vi "Choose_Device.vi"(3 "error in (no error)":errorcluster, 4 "Choose_Device":T1(ring), 5 "Index":i32) -> (0 "error out":errorcluster, 1 "Device_type":T1(ring), 2 "Index_Out":i32)   [LabVIEW 2013, in "FEMTO_LUCI-10.lvlib"]
doc: "This function sets the selected device."
uses:
  FEMTO_LUCI-10.lvlib
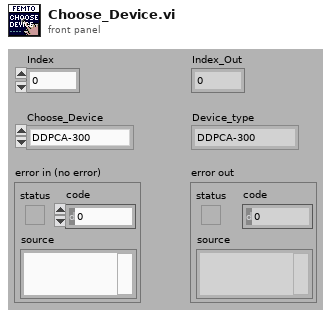
[diagram p1: front panel]
types:
  T1 = enum16{"DDPCA-300", "DLPCA-200", "DHPCA-100", "OE-200", "LIA-MV-150-S", "LIA-MV-150-D", "LIA-MV-200-L", "LIA-MV-200-H", "LIA-MVD-200-L", "LIA-MVD-200-H", "DLPVA-100-BUN-S", "DLPVA-100-BLN-S", "DLPVA-100-B-S", "DLPVA-100-B-D", "DLPVA-100-F-S", "DLPVA-100-F-D", "DHPVA-100", "DHPVA-200", "DUPVA-1-60", "DUPVA-1-70"}
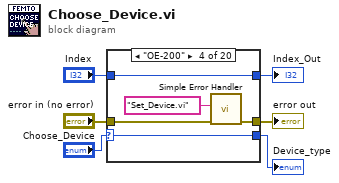
[diagram p0: block diagram]
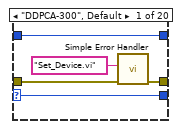
[diagram p2: hidden frame]
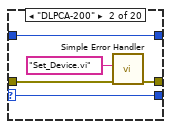
[diagram p3: hidden frame]
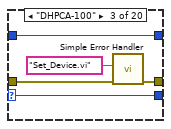
[diagram p4: hidden frame]
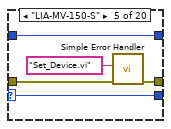
[diagram p5: hidden frame]
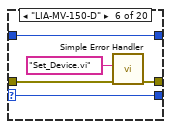
[diagram p6: hidden frame]
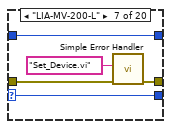
[diagram p7: hidden frame]
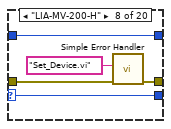
[diagram p8: hidden frame]
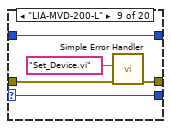
[diagram p9: hidden frame]
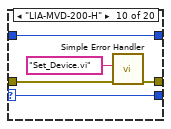
[diagram p10: hidden frame]
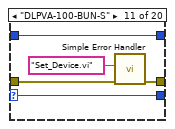
[diagram p11: hidden frame]
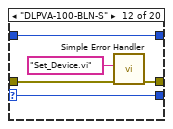
[diagram p12: hidden frame]
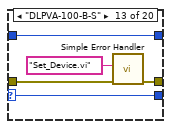
[diagram p13: hidden frame]
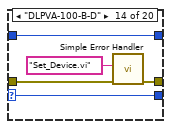
[diagram p14: hidden frame]
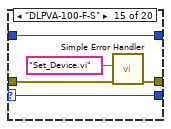
[diagram p15: hidden frame]
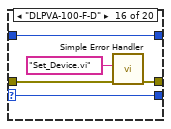
[diagram p16: hidden frame]
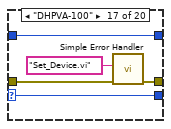
[diagram p17: hidden frame]
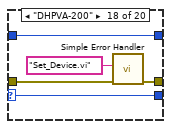
[diagram p18: hidden frame]
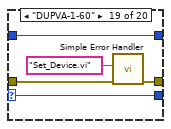
[diagram p19: hidden frame]
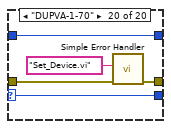
[diagram p20: hidden frame]
diagram:
  n1 = case shown="\"OE-200\"" "Choose_Device" {
    selector: "Choose_Device" -> [w8 w14 w18 w23 w28 w33 w38 w43 w48 w53 w58 w63 w68 w73 w78 w83 w88 w93 w98 w103]
    tunnel: "error in (no error)" -> [w10 w16 w21 w25 w30 w35 w40 w45 w50 w55 w60 w65 w70 w75 w80 w85 w90 w95 w100 w105]
    tunnel: [w9 w15 w20 w24 w29 w34 w39 w44 w49 w54 w59 w64 w69 w74 w79 w84 w89 w94 w99 w104] -> w3
    tunnel: [w8 w14 w18 w23 w28 w33 w38 w43 w48 w53 w58 w63 w68 w73 w78 w83 w88 w93 w98 w103] -> w4
    tunnel: "Index" -> [w7 w12 w17 w22 w27 w32 w37 w42 w47 w52 w57 w62 w67 w72 w77 w82 w87 w92 w97 w102]
    tunnel: [w7 w12 w17 w22 w27 w32 w37 w42 w47 w52 w57 w62 w67 w72 w77 w82 w87 w92 w97 w102] -> w6
    frame "DDPCA-300", Default {
      n2 = call <vilib>:"Simple Error Handler.vi"("error source (\" \")"="Set_Device.vi" ("error source (\" \")"), "error in (no error)"=w10) -> ("error out"=w9:errorcluster)  [unwired: 1 in, 6 out]
    }
    frame "DLPCA-200" {
      n3 = call <vilib>:"Simple Error Handler.vi"("error source (\" \")"="Set_Device.vi" ("error source (\" \")"), "error in (no error)"=w16) -> ("error out"=w15:errorcluster)  [unwired: 1 in, 6 out]
    }
    frame "DHPCA-100" {
      n4 = call <vilib>:"Simple Error Handler.vi"("error source (\" \")"="Set_Device.vi" ("error source (\" \")"), "error in (no error)"=w21) -> ("error out"=w20:errorcluster)  [unwired: 1 in, 6 out]
    }
    frame "OE-200" {
      n5 = call <vilib>:"Simple Error Handler.vi"("error source (\" \")"="Set_Device.vi" ("error source (\" \")"), "error in (no error)"=w25) -> ("error out"=w24:errorcluster)  [unwired: 1 in, 6 out]
    }
    frame "LIA-MV-150-S" {
      n6 = call <vilib>:"Simple Error Handler.vi"("error source (\" \")"="Set_Device.vi" ("error source (\" \")"), "error in (no error)"=w30) -> ("error out"=w29:errorcluster)  [unwired: 1 in, 6 out]
    }
    frame "LIA-MV-150-D" {
      n7 = call <vilib>:"Simple Error Handler.vi"("error source (\" \")"="Set_Device.vi" ("error source (\" \")"), "error in (no error)"=w35) -> ("error out"=w34:errorcluster)  [unwired: 1 in, 6 out]
    }
    frame "LIA-MV-200-L" {
      n8 = call <vilib>:"Simple Error Handler.vi"("error source (\" \")"="Set_Device.vi" ("error source (\" \")"), "error in (no error)"=w40) -> ("error out"=w39:errorcluster)  [unwired: 1 in, 6 out]
    }
    frame "LIA-MV-200-H" {
      n9 = call <vilib>:"Simple Error Handler.vi"("error source (\" \")"="Set_Device.vi" ("error source (\" \")"), "error in (no error)"=w45) -> ("error out"=w44:errorcluster)  [unwired: 1 in, 6 out]
    }
    frame "LIA-MVD-200-L" {
      n10 = call <vilib>:"Simple Error Handler.vi"("error source (\" \")"="Set_Device.vi" ("error source (\" \")"), "error in (no error)"=w50) -> ("error out"=w49:errorcluster)  [unwired: 1 in, 6 out]
    }
    frame "LIA-MVD-200-H" {
      n11 = call <vilib>:"Simple Error Handler.vi"("error source (\" \")"="Set_Device.vi" ("error source (\" \")"), "error in (no error)"=w55) -> ("error out"=w54:errorcluster)  [unwired: 2 in, 5 out]
    }
    frame "DLPVA-100-BUN-S" {
      n12 = call <vilib>:"Simple Error Handler.vi"("error source (\" \")"="Set_Device.vi" ("error source (\" \")"), "error in (no error)"=w60) -> ("error out"=w59:errorcluster)  [unwired: 1 in, 6 out]
    }
    frame "DLPVA-100-BLN-S" {
      n13 = call <vilib>:"Simple Error Handler.vi"("error source (\" \")"="Set_Device.vi" ("error source (\" \")"), "error in (no error)"=w65) -> ("error out"=w64:errorcluster)  [unwired: 1 in, 6 out]
    }
    frame "DLPVA-100-B-S" {
      n14 = call <vilib>:"Simple Error Handler.vi"("error source (\" \")"="Set_Device.vi" ("error source (\" \")"), "error in (no error)"=w70) -> ("error out"=w69:errorcluster)  [unwired: 1 in, 6 out]
    }
    frame "DLPVA-100-B-D" {
      n15 = call <vilib>:"Simple Error Handler.vi"("error source (\" \")"="Set_Device.vi" ("error source (\" \")"), "error in (no error)"=w75) -> ("error out"=w74:errorcluster)  [unwired: 1 in, 6 out]
    }
    frame "DLPVA-100-F-S" {
      n16 = call <vilib>:"Simple Error Handler.vi"("error source (\" \")"="Set_Device.vi" ("error source (\" \")"), "error in (no error)"=w80) -> ("error out"=w79:errorcluster)  [unwired: 1 in, 6 out]
    }
    frame "DLPVA-100-F-D" {
      n17 = call <vilib>:"Simple Error Handler.vi"("error source (\" \")"="Set_Device.vi" ("error source (\" \")"), "error in (no error)"=w85) -> ("error out"=w84:errorcluster)  [unwired: 1 in, 6 out]
    }
    frame "DHPVA-100" {
      n18 = call <vilib>:"Simple Error Handler.vi"("error source (\" \")"="Set_Device.vi" ("error source (\" \")"), "error in (no error)"=w90) -> ("error out"=w89:errorcluster)  [unwired: 1 in, 6 out]
    }
    frame "DHPVA-200" {
      n19 = call <vilib>:"Simple Error Handler.vi"("error source (\" \")"="Set_Device.vi" ("error source (\" \")"), "error in (no error)"=w95) -> ("error out"=w94:errorcluster)  [unwired: 1 in, 6 out]
    }
    frame "DUPVA-1-60" {
      n20 = call <vilib>:"Simple Error Handler.vi"("error source (\" \")"="Set_Device.vi" ("error source (\" \")"), "error in (no error)"=w100) -> ("error out"=w99:errorcluster)  [unwired: 1 in, 6 out]
    }
    frame "DUPVA-1-70" {
      n21 = call <vilib>:"Simple Error Handler.vi"("error source (\" \")"="Set_Device.vi" ("error source (\" \")"), "error in (no error)"=w105) -> ("error out"=w104:errorcluster)  [unwired: 1 in, 6 out]
    }
  }
  "error out" <- w3
  "Device_type" <- w4
  "Index_Out" <- w6
